vi "LDO Button Disable.vi"(7 "UI Refs":T5, 8 "error in (no error)":errorcluster, 10 "PLC Data In":T1, 11 "Queue in":refnum<queue>) -> (0 "error out":errorcluster, 2 "PLC Data Out":T1, 3 "dup Message Queue":refnum<queue>)   [LabVIEW 2020]
uses:
  Message Queue/Message Cluster.ctl
  controls/UI Data.ctl
  Modbus/Modbus PLC Data All.ctl
  Modbus/Modbus FVIR Control.ctl
  Modbus/Modbus LDO Control.ctl
  WritingDataFile/Data to Save.ctl
  Message Queue/Enqueue Message (Single).vi
  Message Queue/Message Queue.lvlib
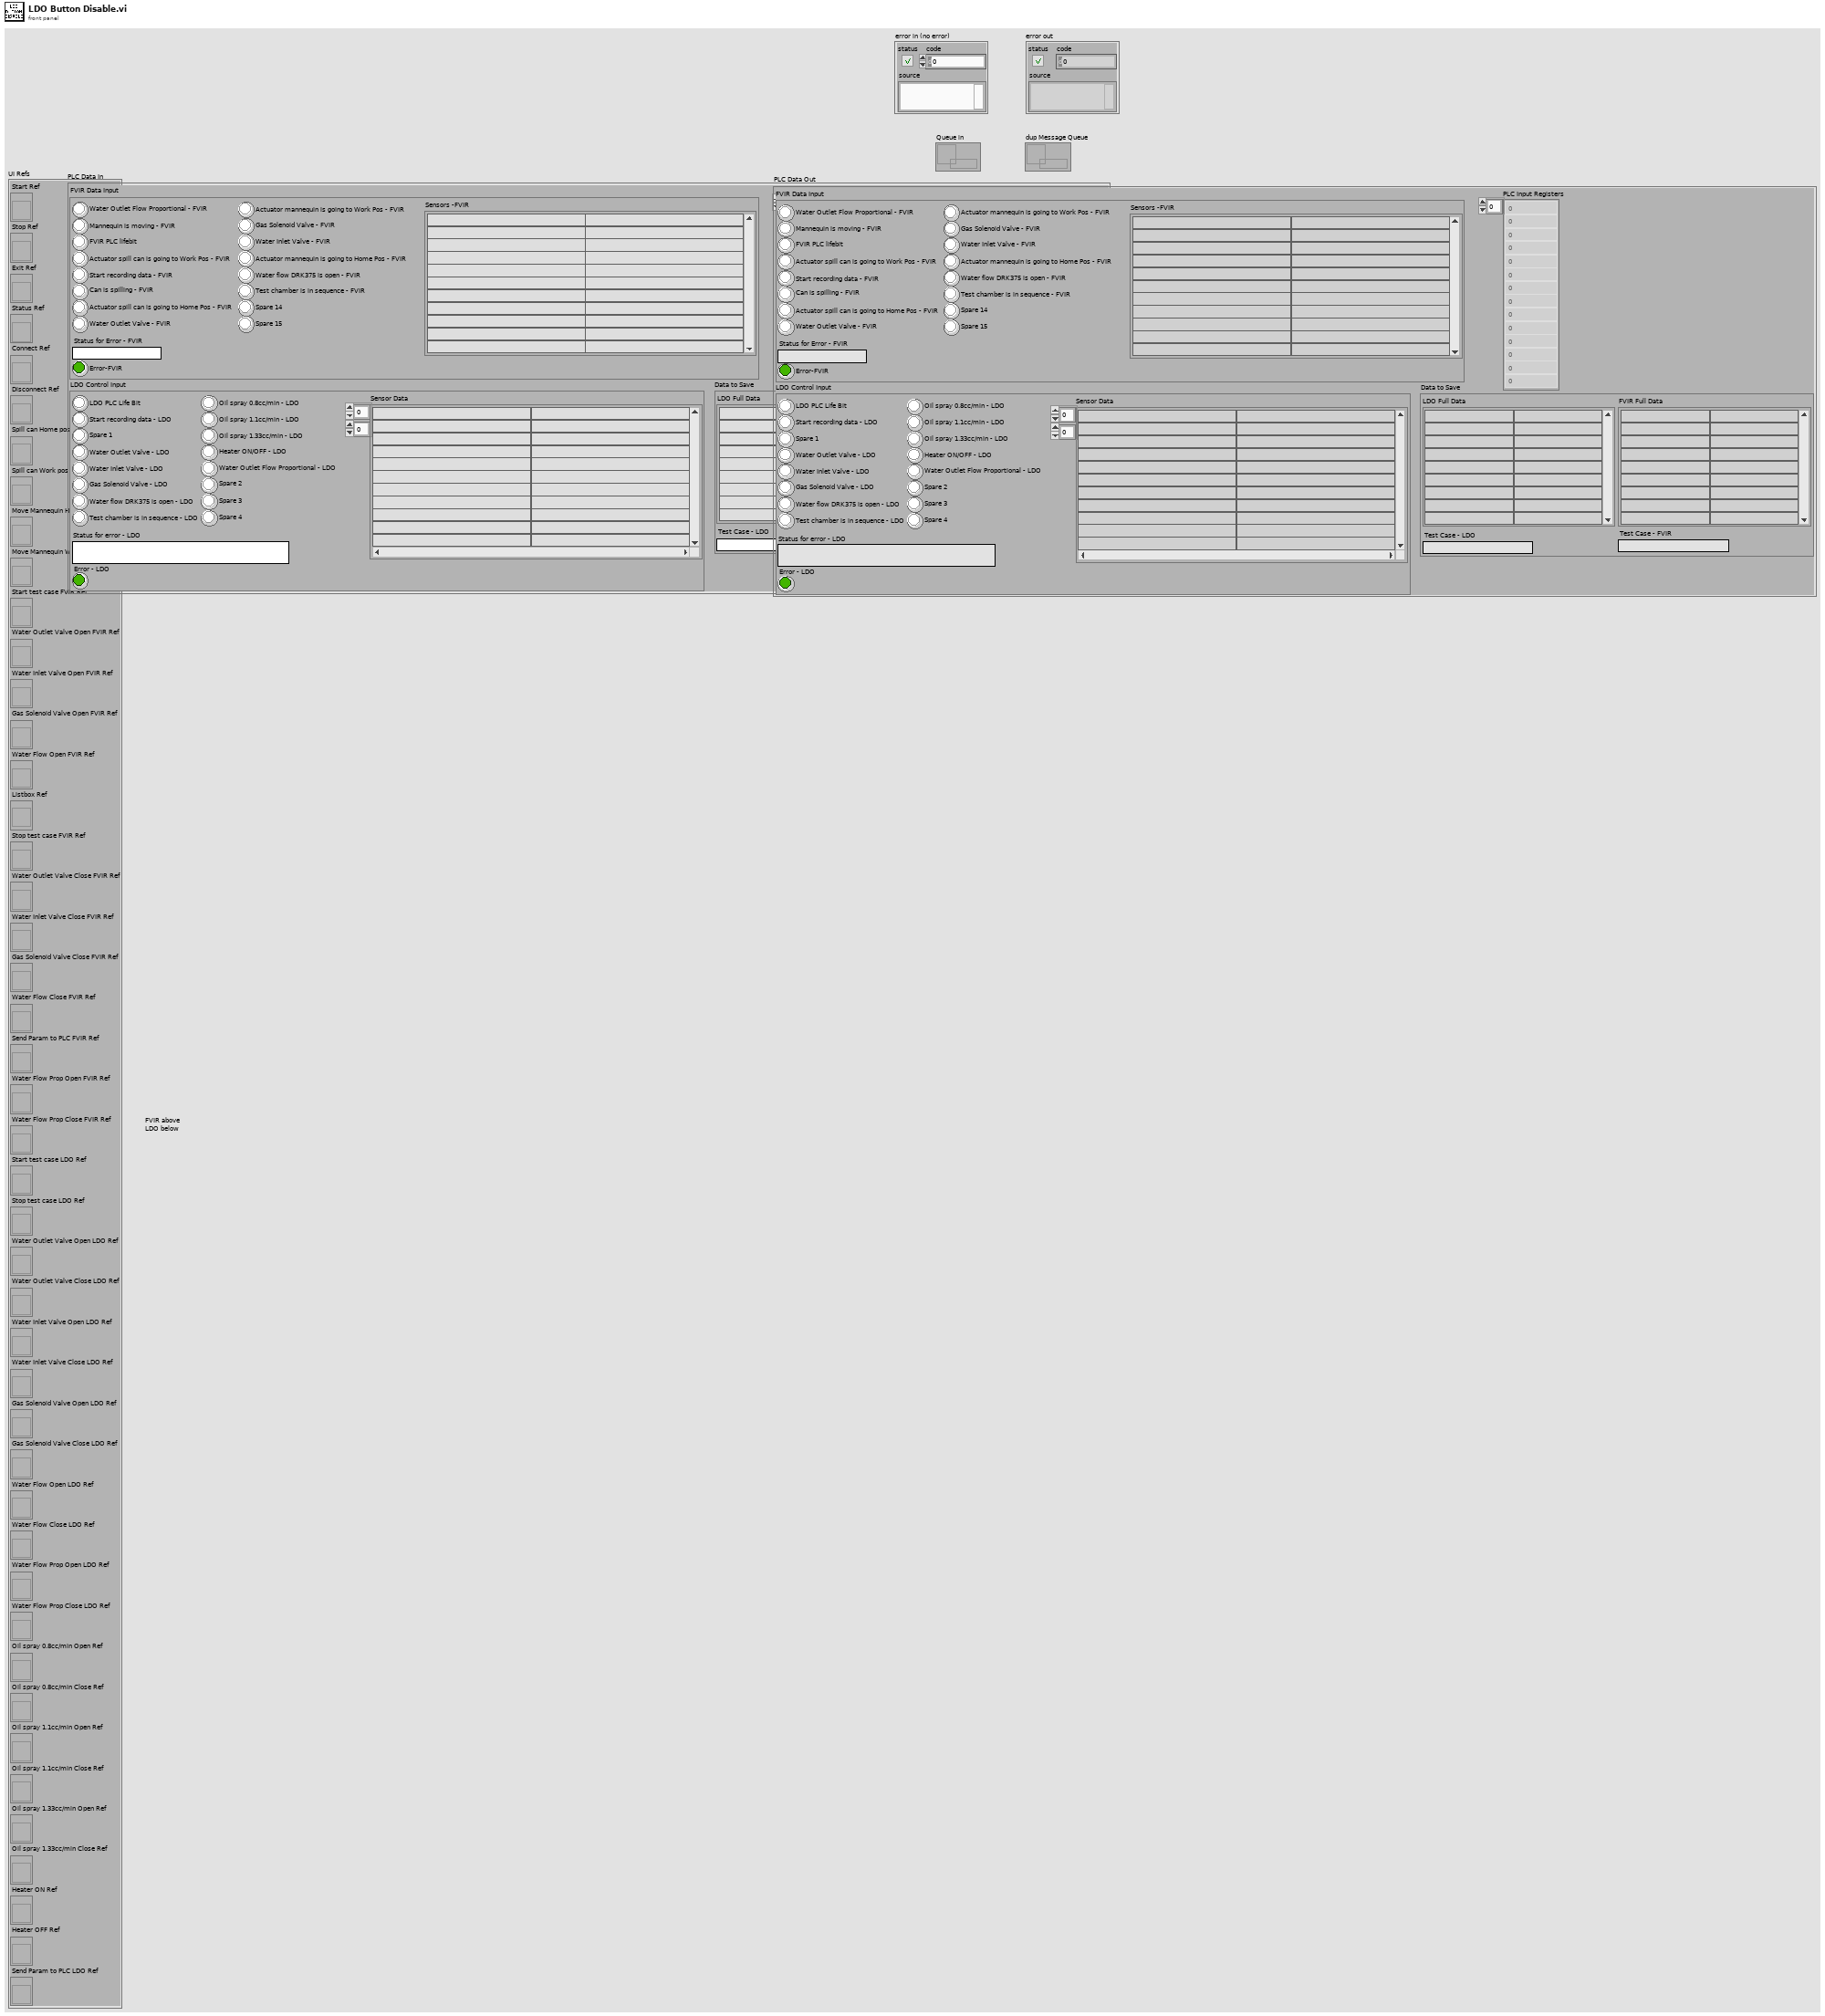
[diagram p1: front panel]
types:
  T1 = typedef "Modbus PLC Data All.ctl" = cluster{"FVIR Data Input":T2, "LDO Control Input":T3, "PLC Input Registers":u16[], "Data to Save":T4}
  T2 = typedef "Modbus FVIR Control.ctl" = cluster{"Spare 15":bool, "Spare 14":bool, "Actuator mannequin is going to Work Pos - FVIR":bool, "Actuator mannequin is going to Home Pos - FVIR":bool, "Test chamber is in sequence - FVIR ":bool, "Water flow DRK375 is open - FVIR":bool, "Gas Solenoid Valve - FVIR":bool, "Water Inlet Valve - FVIR":bool, "Water Outlet Flow Proportional - FVIR":bool, "Start recording data - FVIR":bool, "Actuator spill can is going to Work Pos - FVIR":bool, "Actuator spill can is going to Home Pos - FVIR":bool, "Water Outlet Valve - FVIR":bool, "Can is spilling - FVIR":bool, "Mannequin is moving - FVIR":bool, "FVIR PLC lifebit":bool, "Status for Error - FVIR":string, "Error-FVIR":bool, "Sensors -FVIR":string[][]}
  T3 = typedef "Modbus LDO Control.ctl" = cluster{"LDO PLC Life Bit":bool, "Start recording data - LDO":bool, "Spare 1":bool, "Water Outlet Valve - LDO":bool, "Water Inlet Valve - LDO":bool, "Gas Solenoid Valve - LDO":bool, "Water flow DRK375 is open - LDO":bool, "Test chamber is in sequence - LDO":bool, "Oil spray 0.8cc/min - LDO":bool, "Oil spray 1.1cc/min - LDO":bool, "Oil spray 1.33cc/min - LDO":bool, "Heater ON/OFF - LDO":bool, "Water Outlet Flow Proportional - LDO":bool, "Spare 2":bool, "Spare 3":bool, "Spare 4":bool, "Status for error - LDO":string, "Error - LDO":bool, "Sensor Data":string[][]}
  T4 = typedef "Data to Save.ctl" = cluster{"LDO Full Data":string[][], "FVIR Full Data":string[][], "Test Case - FVIR":string, "Test Case - LDO":string}
  T5 = typedef "UI Data.ctl" = cluster{"Start Ref":refnum<vi>, "Stop Ref":refnum<vi>, "Exit Ref":refnum<vi>, "Status Ref":refnum<vi>, "Connect Ref":refnum<vi>, "Disconnect Ref":refnum<vi>, "Spill can Home pos Ref":refnum<vi>, "Spill can Work pos Ref":refnum<vi>, "Move Mannequin Home pos Ref":refnum<vi>, "Move Mannequin Work pos Ref":refnum<vi>, "Start test case FVIR Ref":refnum<vi>, "Water Outlet Valve Open FVIR Ref":refnum<vi>, "Water Inlet Valve Open FVIR Ref":refnum<vi>, "Gas Solenoid Valve Open FVIR Ref":refnum<vi>, "Water Flow Open FVIR Ref":refnum<vi>, "Listbox Ref":refnum<vi>, "Stop test case FVIR Ref":refnum<vi>, "Water Outlet Valve Close FVIR Ref":refnum<vi>, "Water Inlet Valve Close FVIR Ref":refnum<vi>, "Gas Solenoid Valve Close FVIR Ref":refnum<vi>, "Water Flow Close FVIR Ref":refnum<vi>, "Send Param to PLC FVIR Ref":refnum<vi>, "Water Flow Prop Open FVIR Ref":refnum<vi>, "Water Flow Prop Close FVIR Ref":refnum<vi>, "Start test case LDO Ref":refnum<vi>, "Stop test case LDO Ref":refnum<vi>, "Water Outlet Valve Open LDO Ref":refnum<vi>, "Water Outlet Valve Close LDO Ref":refnum<vi>, "Water Inlet Valve Open LDO Ref":refnum<vi>, "Water Inlet Valve Close LDO Ref":refnum<vi>, "Gas Solenoid Valve Open LDO Ref":refnum<vi>, "Gas Solenoid Valve Close LDO Ref":refnum<vi>, "Water Flow Open LDO Ref":refnum<vi>, "Water Flow Close LDO Ref":refnum<vi>, "Water Flow Prop Open LDO Ref":refnum<vi>, "Water Flow Prop Close LDO Ref":refnum<vi>, "Oil spray 0.8cc/min Open Ref":refnum<vi>, "Oil spray 0.8cc/min Close Ref":refnum<vi>, "Oil spray 1.1cc/min Open Ref":refnum<vi>, "Oil spray 1.1cc/min Close Ref":refnum<vi>, "Oil spray 1.33cc/min Open Ref":refnum<vi>, "Oil spray 1.33cc/min Close Ref":refnum<vi>, "Heater ON Ref":refnum<vi>, "Heater OFF Ref":refnum<vi>, "Send Param to PLC LDO Ref":refnum<vi>}
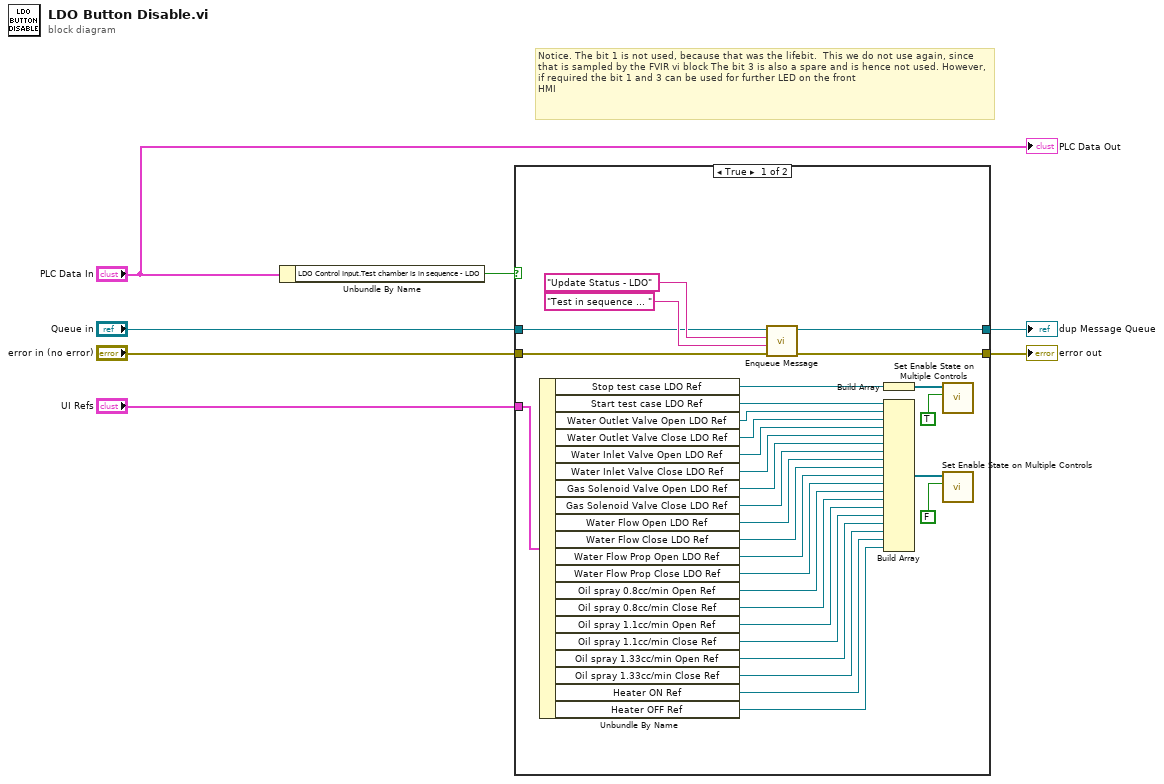
[diagram p0: block diagram]
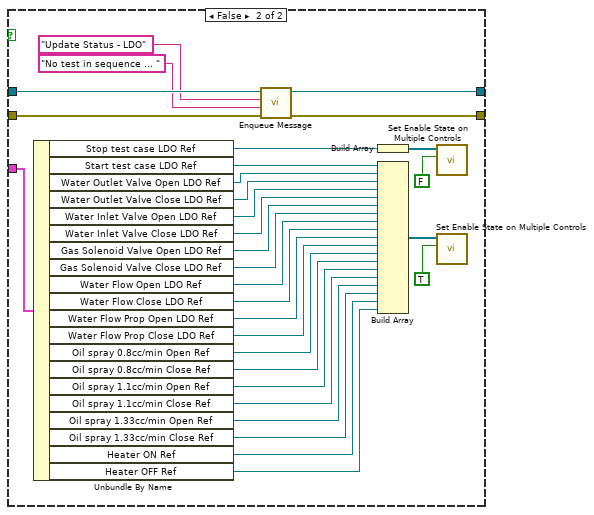
[diagram p2: hidden frame]
diagram:
  # "Notice. The bit 1 is not used, because that was the lifebit.  This we do not use again, since that is sampled by the FVIR vi block The bit 3 is also a spare and is hence not used. However, if required the bit 1 and 3 can be used for further LED on the front \nHMI"
  n1 = Unbundle By Name("PLC Data In") -> ("LDO Control Input.Test chamber is in sequence - LDO"=w1:bool)
  n2 = case shown="True" w1 {
    tunnel: "UI Refs" -> [w38 w69]
    tunnel: "error in (no error)" -> [w13 w44]
    tunnel: [w12 w43] -> w7
    tunnel: "Queue in" -> [w9 w42]
    tunnel: [w8 w39] -> w2
    frame True {
      n3 = Unbundle By Name(w38) -> ("Stop test case LDO Ref"=w36:refnum<vi>, "Start test case LDO Ref"=w35:refnum<vi>, "Water Outlet Valve Open LDO Ref"=w34:refnum<vi>, "Water Outlet Valve Close LDO Ref"=w33:refnum<vi>, "Water Inlet Valve Open LDO Ref"=w32:refnum<vi>, "Water Inlet Valve Close LDO Ref"=w31:refnum<vi>, "Gas Solenoid Valve Open LDO Ref"=w30:refnum<vi>, "Gas Solenoid Valve Close LDO Ref"=w29:refnum<vi>, "Water Flow Open LDO Ref"=w28:refnum<vi>, "Water Flow Close LDO Ref"=w27:refnum<vi>, "Water Flow Prop Open LDO Ref"=w26:refnum<vi>, "Water Flow Prop Close LDO Ref"=w25:refnum<vi>, "Oil spray 0.8cc/min Open Ref"=w24:refnum<vi>, "Oil spray 0.8cc/min Close Ref"=w23:refnum<vi>, "Oil spray 1.1cc/min Open Ref"=w21:refnum<vi>, "Oil spray 1.1cc/min Close Ref"=w20:refnum<vi>, "Oil spray 1.33cc/min Open Ref"=w19:refnum<vi>, "Oil spray 1.33cc/min Close Ref"=w18:refnum<vi>, "Heater ON Ref"=w17:refnum<vi>, "Heater OFF Ref"=w16:refnum<vi>)
      n4 = call-poly "Enqueue Message.vi"("error in (no error)"=w13, "Message Data"="Test in sequence ... " ("Acquiring and Logging..."), "Message"="Update Status - LDO", "Message Queue"=w9) -> ("error out"=w12:errorcluster, "dup Message Queue"=w8:refnum<queue>)  [unwired: 6 in]
      n5 = Build Array(w36) -> (w37:refnum<vi>[])
      n6 = Build Array(w35, w34, w33, w32, w31, w30, w29, w28, w27, w26, w25, w24, w23, w21, w20, w19, w18, w17, w16) -> (w22:refnum<vi>[])
      n7 = call "Set Enable State on Multiple Controls.vi"("Enable?"=TRUE, "Controls"=w37) -> ()  [unwired: 10 in]
      n8 = call "Set Enable State on Multiple Controls.vi"("Enable?"=FALSE, "Controls"=w22) -> ()  [unwired: 10 in]
    }
    frame False {
      n9 = Unbundle By Name(w69) -> ("Stop test case LDO Ref"=w67:refnum<vi>, "Start test case LDO Ref"=w66:refnum<vi>, "Water Outlet Valve Open LDO Ref"=w65:refnum<vi>, "Water Outlet Valve Close LDO Ref"=w64:refnum<vi>, "Water Inlet Valve Open LDO Ref"=w63:refnum<vi>, "Water Inlet Valve Close LDO Ref"=w62:refnum<vi>, "Gas Solenoid Valve Open LDO Ref"=w61:refnum<vi>, "Gas Solenoid Valve Close LDO Ref"=w60:refnum<vi>, "Water Flow Open LDO Ref"=w59:refnum<vi>, "Water Flow Close LDO Ref"=w58:refnum<vi>, "Water Flow Prop Open LDO Ref"=w57:refnum<vi>, "Water Flow Prop Close LDO Ref"=w56:refnum<vi>, "Oil spray 0.8cc/min Open Ref"=w55:refnum<vi>, "Oil spray 0.8cc/min Close Ref"=w54:refnum<vi>, "Oil spray 1.1cc/min Open Ref"=w52:refnum<vi>, "Oil spray 1.1cc/min Close Ref"=w51:refnum<vi>, "Oil spray 1.33cc/min Open Ref"=w50:refnum<vi>, "Oil spray 1.33cc/min Close Ref"=w49:refnum<vi>, "Heater ON Ref"=w48:refnum<vi>, "Heater OFF Ref"=w47:refnum<vi>)
      n10 = call-poly "Enqueue Message.vi"("error in (no error)"=w44, "Message Data"="No test in sequence ... " ("Acquiring and Logging..."), "Message"="Update Status - LDO", "Message Queue"=w42) -> ("error out"=w43:errorcluster, "dup Message Queue"=w39:refnum<queue>)  [unwired: 6 in]
      n11 = Build Array(w67) -> (w68:refnum<vi>[])
      n12 = Build Array(w66, w65, w64, w63, w62, w61, w60, w59, w58, w57, w56, w55, w54, w52, w51, w50, w49, w48, w47) -> (w53:refnum<vi>[])
      n13 = call "Set Enable State on Multiple Controls.vi"("Enable?"=FALSE, "Controls"=w68) -> ()  [unwired: 10 in]
      n14 = call "Set Enable State on Multiple Controls.vi"("Enable?"=TRUE, "Controls"=w53) -> ()  [unwired: 10 in]
    }
  }
  "error out" <- w7
  "dup Message Queue" <- w2
  "PLC Data Out" <- "PLC Data In"
